vi "UI-BaseParamSet.vi"(8 "error in (no error)":errorcluster caption="错误输入（无错误）") -> (0 "error out":errorcluster caption="错误输出")   [LabVIEW 2017]
uses:
  Picture/SaveButtom.ctl
  Global System.vi
panel:
  in  "Program Update":bool
  in  "Machine Paramter Save Buttom":T1
  out "system time":string
  in  "选项卡控件":enum32{"BaseParamSet", "OtherParamSet"}(tab)
  in  "条码扫描周期":string
  in  "LoadProgram":string(combo)
  in  "BaseParams Save Buttom":T1
  in  "参数B":string
  in  "参数K":string
  in  "校正像素值":string
  in  "Tolerance Params Save":T1
  in  "单位距离":string
  # "秒"
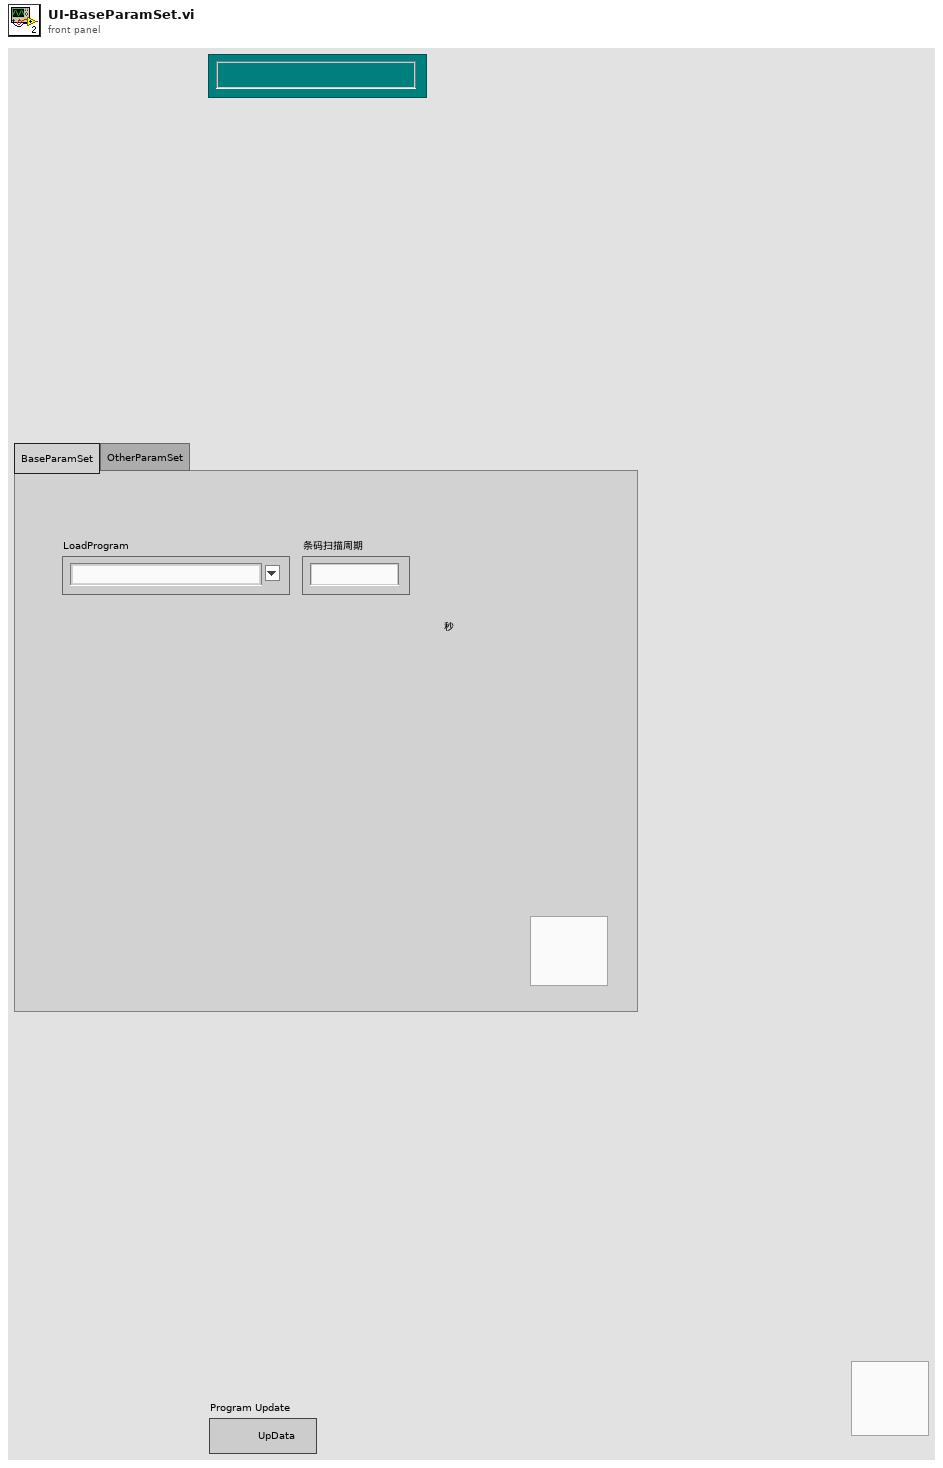
[diagram p1: front panel]
types:
  T1 = typedef "SaveButtom.ctl" = bool
  T2 = cluster{"master data":string, "priority":u16, "secondary data":string[]}
  T3 = cluster{"case name":string[], "queue array":refnum<queue>[]}
  T4 = cluster{"导通气缸上位置":bool, "导通气缸下位置\n":bool, "工位一料到位信号":bool, "工位二料到位信号":bool, "工位三料到位信号":bool, "转盘到位信号":bool, "凸轮感应信号":bool, "导通信号":bool, "真空":bool, "备用":bool, "备用":bool, "备用":bool, "备用":bool, "备用":bool, "备用":bool, "备用":bool, "备用":bool, "备用":bool, "备用":bool, "备用":bool, "备用":bool, "备用":bool, "备用":bool, "备用":bool}
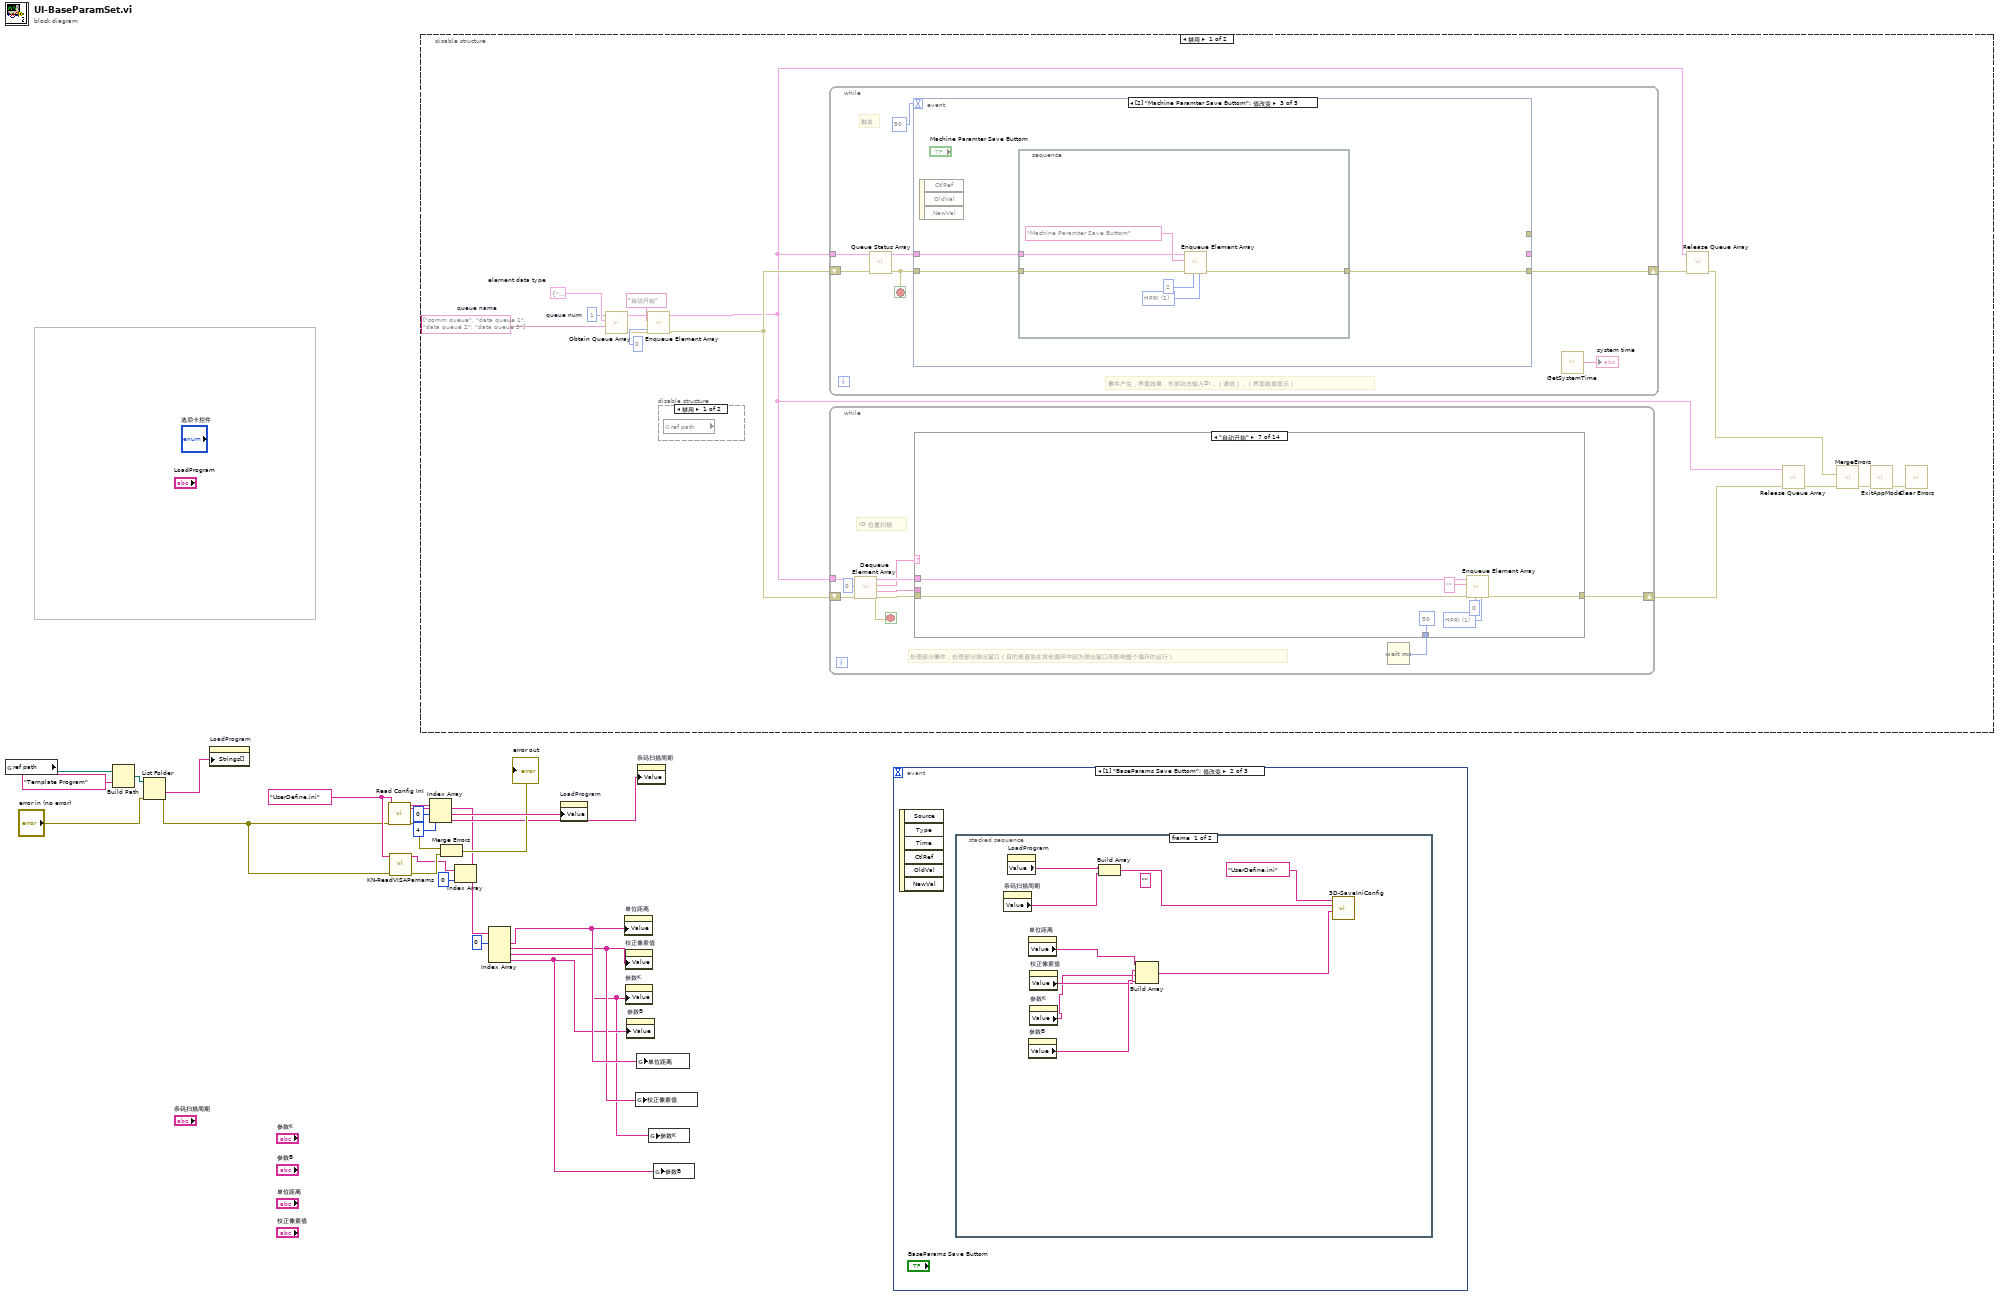
[diagram p0: block diagram]
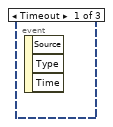
[diagram p2: hidden frame]
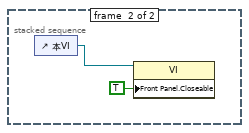
[diagram p3: hidden frame]
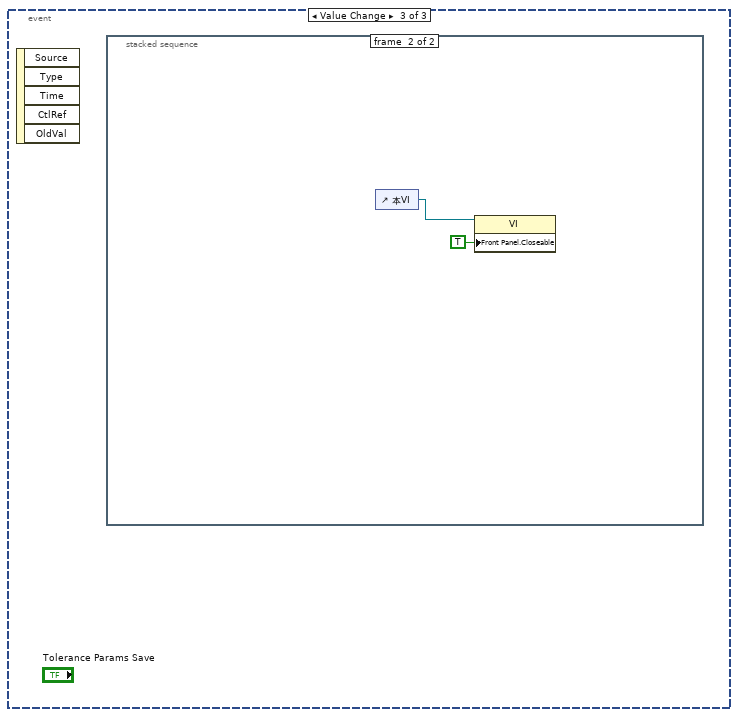
[diagram p4: hidden frame]
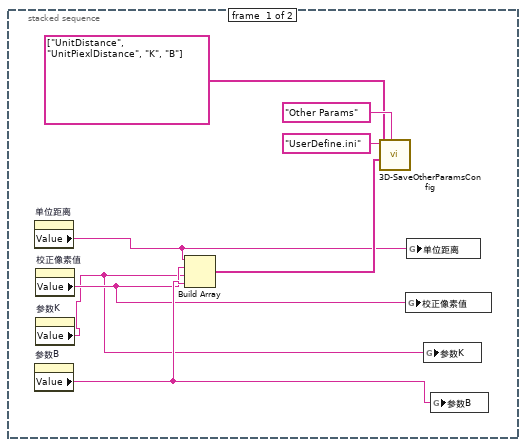
[diagram p5: hidden frame]
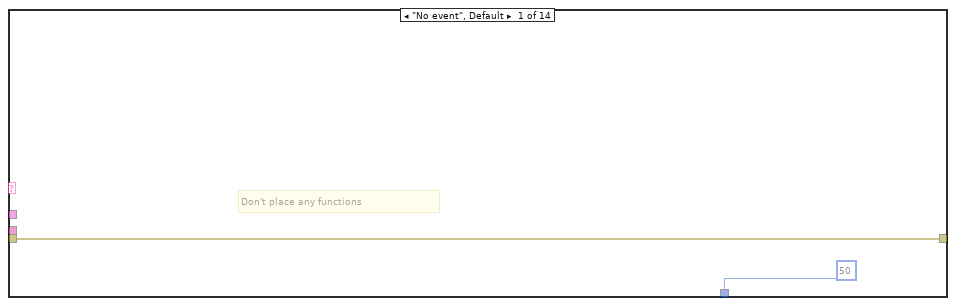
[diagram p7: hidden frame]
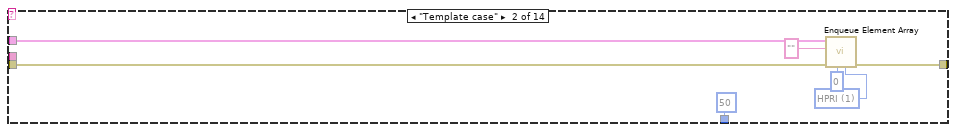
[diagram p8: hidden frame]
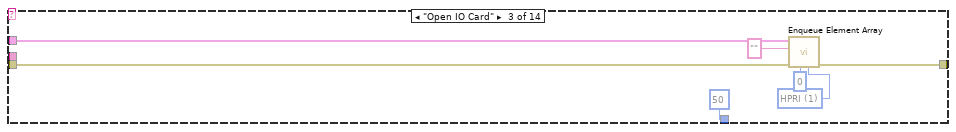
[diagram p9: hidden frame]
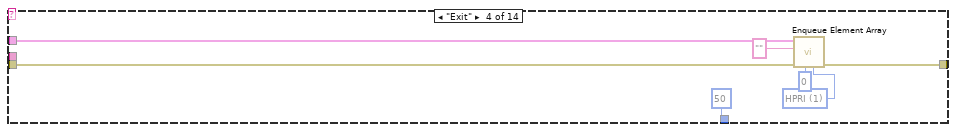
[diagram p10: hidden frame]
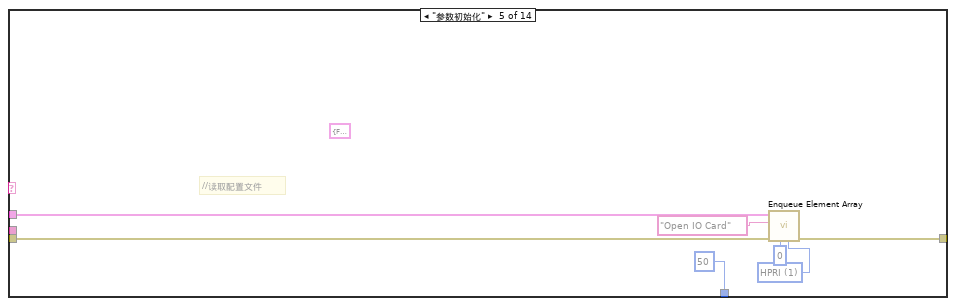
[diagram p11: hidden frame]
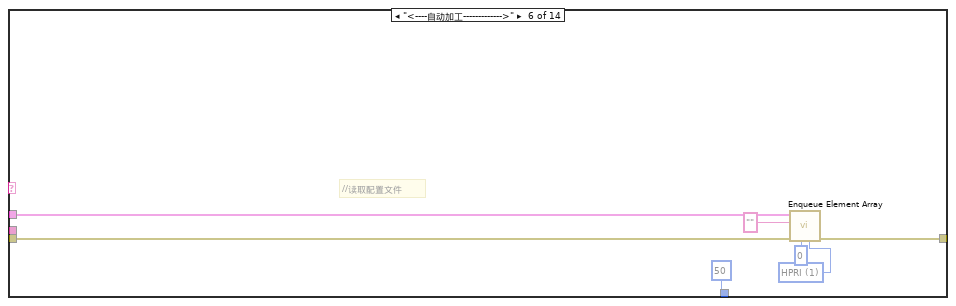
[diagram p12: hidden frame]
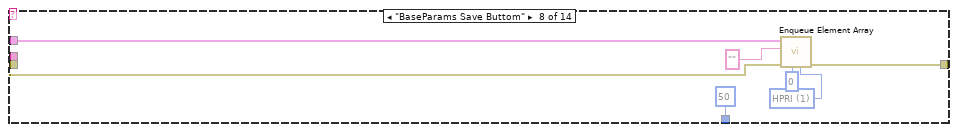
[diagram p13: hidden frame]
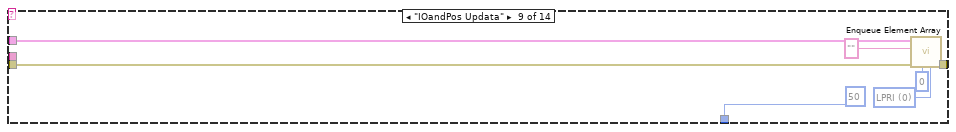
[diagram p14: hidden frame]
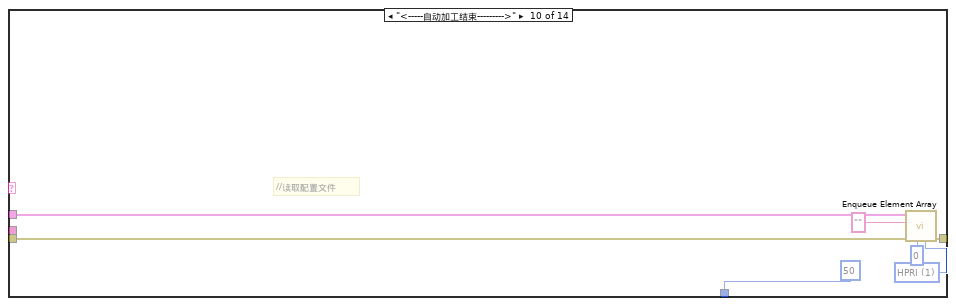
[diagram p15: hidden frame]
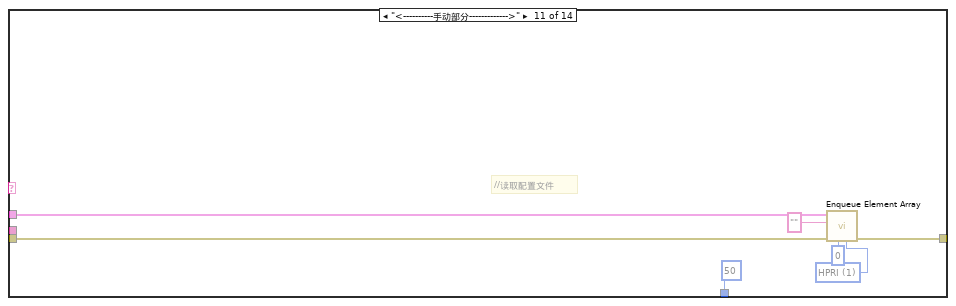
[diagram p16: hidden frame]
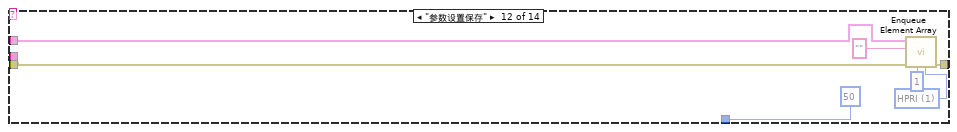
[diagram p17: hidden frame]
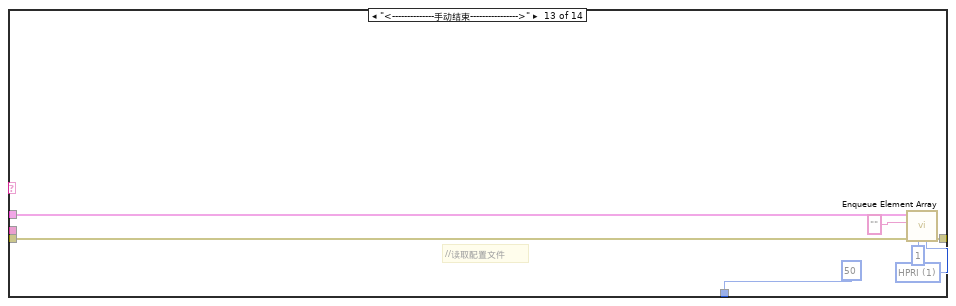
[diagram p18: hidden frame]
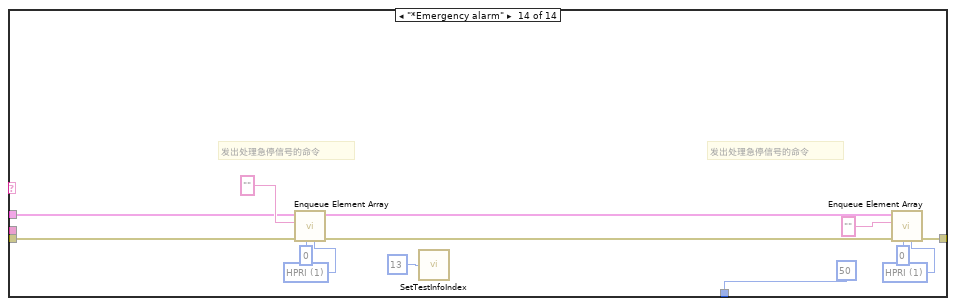
[diagram p19: hidden frame]
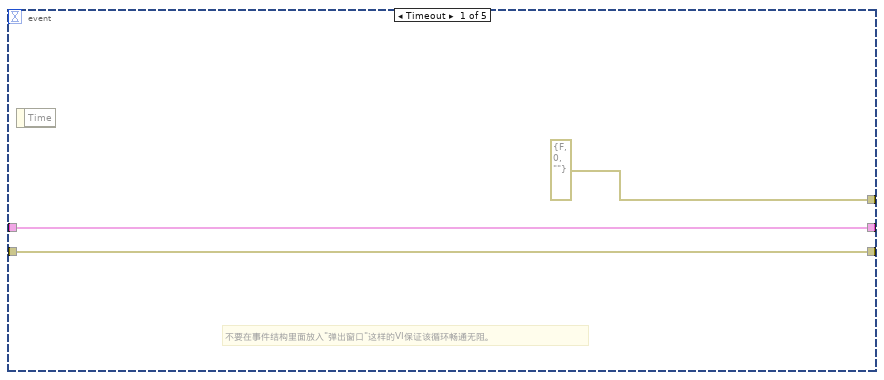
[diagram p20: hidden frame]
diagram:
  w20 = "UserDefine.ini" ("名称或相对路径")
  n1 = global read "Global System.vi" "ref path"() -> (w14:path)
  n2 = Build Path(base path=w14, name or relative path="Template Program" ("名称或相对路径")) -> (appended path=w12:path)
  n3 = List Folder(path=w12, error in="error in (no error)") -> (folder names=w11:string[], error out=w9:errorcluster)  [unwired: 2 in, 2 out]
  n4 = property on="LoadProgram" class="CmbBox"("Strings[]"=w11) -> ()  [unwired: 2 in, 2 out]
  n5 = call "Read Config InI.vi"("名称或相对路径"=w20, "error in (no error)"=w9) -> ("ParamSet"=w22:string[], "Other Params"=w6:string[], "error out"=w19:errorcluster)  [unwired: 13 in, 2 out]
  n6 = call "KN-ReadVISAPamams.vi"("名称或相对路径"=w20, "error in (no error)"=w9) -> ("VISA1 Param"=w16:string[], "error out"=w18:errorcluster)  [unwired: 12 in]
  n7 = disable-structure shown="禁用" {
    frame Disabled {
      w37 = 1  # queue num
      w38 = T2 {"master data"="", "priority"=0, "secondary data"=[]}  # element data type
      w36 = string[] ["comm queue", "data queue 1", "data queue 2", "data queue 3"]  # queue name
      n8 = call "Obtain Queue Array.vi"("queue name"=w36, "element data type"=w38, "queue num"=w37) -> ("error out"=w32:errorcluster, "queue out"=w33:T3)  [unwired: 2 in, 1 out]
      n9 = call "Enqueue Element Array.vi"("queue index"=0, "error in"=w32, "master data"="自动开始", "queue in"=w33) -> ("error out"=w26:errorcluster, "queue out"=w24:T3)  [unwired: 6 in]
      n10 = disable-structure shown="禁用" {
        frame Disabled {
          n11 = global read "Global System.vi" "ref path"() -> ()  [unwired: 1 out]
        }
        frame Enabled {
        }
      }
      n12 = while {
        shift-right: [w147] -> w27
        shift-left: w26 -> [w150]
        tunnel: w24 -> [w152]
        stop <- w148 stop-if-true
        # "触发"
        # "事件产生，界面效果，外部状态输入DI，（通信），（界面数据显示）"
        n13 = call "Queue Status Array.vi"("error in (no error)"=w150, "queue in"=w152) -> ("error out"=w148:errorcluster, "queue out"=w149:T3)  [unwired: 4 in]
        n14 = event shown="[2] \"Machine Paramter Save Buttom\": 值改变" {
          selector: _ -> [_ _ _ _ _]
          dyn-events: _ -> [_ _ _ _ _]
          timeout: 50 -> [_ _ _ _ _]
          tunnel: [errorcluster {"status"=FALSE, "code"=0, "source"=""} ("error out") _ _ _ _] -> _
          tunnel: w149 -> [w155 w163 w167 w176 w188]
          tunnel: w148 -> [w154 w162 w166 w175 w187]
          tunnel: [w154 w161 w165 w174 w186] -> w147
          tunnel: [w155 w160 _ _ _] -> _
          event Timeout {
            # "不要在事件结构里面放入\"弹出窗口\"这样的VI保证该循环畅通无阻。"
            n15 = event-data() -> ()  [unwired: 1 in, 1 out]
          }
          event Panel Close? {
            w158 = u16 1 items=["HPRI"=1, "LPRI"=0] ("priority")
            n16 = event-data() -> ()  [unwired: 1 in, 4 out]
            n17 = call "Enqueue Element Array.vi"("priority"=w158, "queue index"=0, "error in"=w162, "master data"="*Exit application", "queue in"=w163) -> ("error out"=w161:errorcluster, "queue out"=w160:T3)  [unwired: 5 in]
            n18 = event-data("Discard?"=TRUE) -> ()  [unwired: 1 in, 1 out]
          }
          event Value Change {
            n19 = event-data() -> ()  [unwired: 1 in, 3 out]
            n20 = stacked-sequence {
              tunnel: w167 -> [w170]
              tunnel: w166 -> [w169]
              tunnel: [w168] -> w165
              frame #0 {
                w172 = u16 1 items=["HPRI"=1, "LPRI"=0] ("priority")
                n21 = call "Enqueue Element Array.vi"("priority"=w172, "queue index"=2, "error in"=w169, "master data"="Machine Paramter Save Buttom", "queue in"=w170) -> ("error out"=w168:errorcluster)  [unwired: 5 in, 1 out]
              }
            }
          }
          event "Program Update": Value Change {
            n22 = event-data() -> ()  [unwired: 1 in, 6 out]
            n23 = stacked-sequence {
              tunnel: w176 -> [w179]
              tunnel: w175 -> [w178]
              tunnel: [w177] -> w174
              frame #0 {
                w181 = u16 1 items=["HPRI"=1, "LPRI"=0] ("priority")
                n24 = call "Enqueue Element Array.vi"("priority"=w181, "queue index"=2, "error in"=w178, "master data"="Program Update", "queue in"=w179) -> ("error out"=w177:errorcluster)  [unwired: 5 in, 1 out]
              }
            }
          }
          event Value Change {
            w184 = u16 1 items=["HPRI"=1, "LPRI"=0] ("priority")
            n25 = event-data() -> ()  [unwired: 1 in, 3 out]
            n26 = call "Enqueue Element Array.vi"("priority"=w184, "queue index"=0, "error in"=w187, "master data"="BaseParams Save Buttom", "queue in"=w188) -> ("error out"=w186:errorcluster)  [unwired: 5 in, 1 out]
          }
        }
        n27 = call "GetSystemTime.vi"() -> ("date/time string"=→"system time":string)  [unwired: 7 in]
      }
      n28 = while {
        shift-right: [w47] -> w25
        shift-left: w26 -> [w45]
        tunnel: w24 -> [w41]
        stop <- w40 stop-if-true
        # "IO 位置扫描"
        # "处理部分事件；处理部分弹出窗口（目的是避免在其他循环中因为弹出窗口而影响整个循环的运行）"
        n29 = call "Dequeue Element Array.vi"("queue in"=w41, "queue index"=0, "error in"=w45) -> ("queue out"=w44:T3, "master data"=w43:string, "secondary data"=w42:string[], "error out"=w40:errorcluster)  [unwired: 2 in, 1 out]
        n30 = case shown="\"自动开始\"" w43 {
          tunnel: w44 -> [_ w55 w62 w69 w76 w83 w85 w97 w104 w111 w118 w125 w132 w138]
          tunnel: w40 -> [w49 w52 w59 w66 w73 w80 w88 w94 w99 w108 w115 w122 w129 w135]
          tunnel: [w49 w54 w61 w68 w75 w82 w90 w96 w103 w110 w117 w124 w131 w145] -> w47
          tunnel: [50 50 50 50 50 50 50 50 50 50 50 50 50 50] -> w46
          tunnel: w42 -> [_ _ _ _ _ _ _ _ _ _ _ _ _ _]
          frame "No event", Default {
            # "Don't place any functions"
          }
          frame "Template case" {
            w50 = u16 1 items=["HPRI"=1, "LPRI"=0] ("priority")
            n31 = call "Enqueue Element Array.vi"("priority"=w50, "queue index"=0, "error in"=w52, "master data"="" ("Element 1"), "queue in"=w55) -> ("error out"=w54:errorcluster)  [unwired: 5 in, 1 out]
          }
          frame "Open IO Card" {
            w57 = u16 1 items=["HPRI"=1, "LPRI"=0] ("priority")
            n32 = call "Enqueue Element Array.vi"("priority"=w57, "queue index"=0, "error in"=w59, "master data"="" ("Element 1"), "queue in"=w62) -> ("error out"=w61:errorcluster)  [unwired: 5 in, 1 out]
          }
          frame "Exit" {
            w64 = u16 1 items=["HPRI"=1, "LPRI"=0] ("priority")
            n33 = call "Enqueue Element Array.vi"("priority"=w64, "queue index"=0, "error in"=w66, "master data"="" ("Element 1"), "queue in"=w69) -> ("error out"=w68:errorcluster)  [unwired: 5 in, 1 out]
          }
          frame "参数初始化" {
            (unwired) T4 {"导通气缸上位置"=FALSE, "导通气缸下位置\n"=FALSE, "工位一料到位信号"=FALSE, "工位二料到位信号"=FALSE, "工位三料到位信号"=FALSE, "转盘到位信号"=FALSE, "凸轮感应信号"=FALSE, "导通信号"=FALSE, "真空"=FALSE, "备用"=FALSE, "备用"=FALSE, "备用"=FALSE, "备用"=FALSE, "备用"=FALSE, "备用"=FALSE, "备用"=FALSE, "备用"=FALSE, "备用"=FALSE, "备用"=FALSE, "备用"=FALSE, "备用"=FALSE, "备用"=FALSE, "备用"=FALSE, "备用"=FALSE} ("7230 设备DO")
            w71 = u16 1 items=["HPRI"=1, "LPRI"=0] ("priority")
            # "//读取配置文件"
            n34 = call "Enqueue Element Array.vi"("priority"=w71, "queue index"=0, "error in"=w73, "master data"="Open IO Card" ("Element 1"), "queue in"=w76) -> ("error out"=w75:errorcluster)  [unwired: 5 in, 1 out]
          }
          frame "<----自动加工------------->" {
            w78 = u16 1 items=["HPRI"=1, "LPRI"=0] ("priority")
            # "//读取配置文件"
            n35 = call "Enqueue Element Array.vi"("priority"=w78, "queue index"=0, "error in"=w80, "master data"="" ("Element 1"), "queue in"=w83) -> ("error out"=w82:errorcluster)  [unwired: 5 in, 1 out]
          }
          frame "自动开始" {
            w86 = u16 1 items=["HPRI"=1, "LPRI"=0] ("priority")
            n36 = call "Enqueue Element Array.vi"("priority"=w86, "queue index"=0, "error in"=w88, "master data"="" ("Element 1"), "queue in"=w85) -> ("error out"=w90:errorcluster)  [unwired: 5 in, 1 out]
          }
          frame "BaseParams Save Buttom" {
            w92 = u16 1 items=["HPRI"=1, "LPRI"=0] ("priority")
            n37 = call "Enqueue Element Array.vi"("priority"=w92, "queue index"=0, "error in"=w94, "master data"="" ("Element 1"), "queue in"=w97) -> ("error out"=w96:errorcluster)  [unwired: 5 in, 1 out]
          }
          frame "IOandPos Updata" {
            w101 = u16 0 items=["HPRI"=1, "LPRI"=0] ("priority")
            n38 = call "Enqueue Element Array.vi"("priority"=w101, "queue index"=0, "error in"=w99, "master data"="", "queue in"=w104) -> ("error out"=w103:errorcluster)  [unwired: 5 in, 1 out]
          }
          frame "<-----自动加工结束--------->" {
            w106 = u16 1 items=["HPRI"=1, "LPRI"=0] ("priority")
            # "//读取配置文件"
            n39 = call "Enqueue Element Array.vi"("priority"=w106, "queue index"=0, "error in"=w108, "master data"="" ("Element 1"), "queue in"=w111) -> ("error out"=w110:errorcluster)  [unwired: 5 in, 1 out]
          }
          frame "<----------手动部分------------->" {
            w113 = u16 1 items=["HPRI"=1, "LPRI"=0] ("priority")
            # "//读取配置文件"
            n40 = call "Enqueue Element Array.vi"("priority"=w113, "queue index"=0, "error in"=w115, "master data"="" ("Element 1"), "queue in"=w118) -> ("error out"=w117:errorcluster)  [unwired: 5 in, 1 out]
          }
          frame "参数设置保存" {
            w120 = u16 1 items=["HPRI"=1, "LPRI"=0] ("priority")
            n41 = call "Enqueue Element Array.vi"("priority"=w120, "queue index"=1, "error in"=w122, "master data"="" ("Element 1"), "queue in"=w125) -> ("error out"=w124:errorcluster)  [unwired: 5 in, 1 out]
          }
          frame "<--------------手动结束---------------->" {
            w127 = u16 1 items=["HPRI"=1, "LPRI"=0] ("priority")
            # "//读取配置文件"
            n42 = call "Enqueue Element Array.vi"("priority"=w127, "queue index"=1, "error in"=w129, "master data"="" ("Element 1"), "queue in"=w132) -> ("error out"=w131:errorcluster)  [unwired: 5 in, 1 out]
          }
          frame "*Emergency alarm" {
            w141 = u16 1 items=["HPRI"=1, "LPRI"=0] ("priority")
            w142 = u16 1 items=["HPRI"=1, "LPRI"=0] ("priority")
            # "发出处理急停信号的命令"
            # "发出处理急停信号的命令"
            n43 = call "Enqueue Element Array.vi"("priority"=w141, "queue index"=0, "error in"=w135, "master data"="" ("Element 1"), "queue in"=w138) -> ("error out"=w136:errorcluster, "queue out"=w137:T3)  [unwired: 5 in]
            n44 = call "SetTestInfoIndex.vi"("test info index"=13) -> ()
            n45 = call "Enqueue Element Array.vi"("priority"=w142, "queue index"=0, "error in"=w136, "master data"="" ("Element 1"), "queue in"=w137) -> ("error out"=w145:errorcluster)  [unwired: 5 in, 1 out]
          }
        }
        n46 = Wait (ms)(milliseconds to wait=w46) -> ()  [unwired: 1 out]
      }
      n47 = call "Release Queue Array.vi"("error in"=w27, "queue in"=w24) -> ("error out"=w29:errorcluster)  [unwired: 2 in, 3 out]
      n48 = call "Release Queue Array.vi"("error in"=w25, "queue in"=w24) -> ("error out"=w31:errorcluster)  [unwired: 2 in, 3 out]
      n49 = call "MergeErrors.vi"("error in 2 (no error)"=w29, "error in 4 (no error)"=w31) -> ("error out"=w30:errorcluster)  [unwired: 6 in]
      n50 = call "ExitAppMode.vi"("error in (no error)"=w30) -> ("error out"=w28:errorcluster)  [unwired: 10 in]
      n51 = call <vilib>:"Clear Errors.vi"("error in (no error)"=w28) -> ()  [unwired: 5 in, 2 out]
    }
    frame Enabled {
    }
  }
  n52 = Index Array(array=w22, index #1=0 ("索引"), index #2=4 ("索引")) -> (element #1=w21:string, element #2=w7:string)
  n53 = Merge Errors(w19, w18) -> (→"error out":errorcluster)
  n54 = Index Array(array=w16, index=0 ("索引")) -> ()  [unwired: 1 out]
  n55 = Index Array(array=w6, index #1=0 ("索引")) -> (element #1=w4:string, element #2=w3:string, element #3=w1:string, element #4=w2:string)  [unwired: 3 in]
  n56 = property on="LoadProgram" class="CmbBox"("Value"=w21) -> ()  [unwired: 2 in, 2 out]
  n57 = property on="单位距离" class="Str"("Value"=w4) -> ()  [unwired: 2 in, 2 out]
  n58 = property on="校正像素值" class="Str"("Value"=w3) -> ()  [unwired: 2 in, 2 out]
  n59 = property on="参数K" class="Str"("Value"=w1) -> ()  [unwired: 2 in, 2 out]
  n60 = property on="参数B" class="Str"("Value"=w2) -> ()  [unwired: 2 in, 2 out]
  n61 = global write "Global System.vi" "校正像素值"(w3) -> ()
  n62 = global write "Global System.vi" "单位距离"(w4) -> ()
  n63 = property on="条码扫描周期" class="Str"("Value"=w7) -> ()  [unwired: 2 in, 2 out]
  n64 = global write "Global System.vi" "参数K"(w1) -> ()
  n65 = global write "Global System.vi" "参数B"(w2) -> ()
  n66 = event shown="[1] \"BaseParams Save Buttom\": 值改变" {
    selector: _ -> [_ _ _]
    dyn-events: _ -> [_ _ _]
    timeout: _ -> [_ _ _]
    event Timeout {
      n67 = event-data() -> ()  [unwired: 1 in, 3 out]
    }
    event Value Change {
      n68 = event-data() -> ()  [unwired: 1 in, 6 out]
      n69 = stacked-sequence {
        frame #0 {
          (unwired) ""
          n70 = property on="条码扫描周期" class="Str"() -> ("Value"=w194:string)  [unwired: 2 in, 2 out]
          n71 = property on="LoadProgram" class="CmbBox"() -> ("Value"=w196:string)  [unwired: 2 in, 2 out]
          n72 = property on="单位距离" class="Str"() -> ("Value"=w193:string)  [unwired: 2 in, 2 out]
          n73 = property on="参数B" class="Str"() -> ("Value"=w192:string)  [unwired: 2 in, 2 out]
          n74 = property on="校正像素值" class="Str"() -> ("Value"=w191:string)  [unwired: 2 in, 2 out]
          n75 = property on="参数K" class="Str"() -> ("Value"=w190:string)  [unwired: 2 in, 2 out]
          n76 = Build Array(w196, w194) -> (w195:string[])
          n77 = Build Array(w193, w191, w190, w192) -> (w189:string[])
          n78 = call "3D-SaveIniConfig.vi"("VISA1"=w189, "Inputs_BaseParam"=w195, "名称或相对路径"="UserDefine.ini") -> ()  [unwired: 9 in]
        }
        frame #1 {
          n79 = control-ref of="本VI"() -> (w199:refnum<vi>)
          n80 = property class="VI"(reference=w199, "Front Panel.Closeable"=TRUE ("前面板窗口:可关闭")) -> ()  [unwired: 1 in, 2 out]
        }
      }
    }
    event Value Change {
      n81 = event-data() -> ()  [unwired: 1 in, 5 out]
      n82 = stacked-sequence {
        frame #0 {
          n83 = property on="单位距离" class="Str"() -> ("Value"=w203:string)  [unwired: 2 in, 2 out]
          n84 = property on="参数B" class="Str"() -> ("Value"=w202:string)  [unwired: 2 in, 2 out]
          n85 = property on="校正像素值" class="Str"() -> ("Value"=w201:string)  [unwired: 2 in, 2 out]
          n86 = property on="参数K" class="Str"() -> ("Value"=w200:string)  [unwired: 2 in, 2 out]
          n87 = Build Array(w203, w201, w200, w202) -> (w204:string[])
          n88 = call "3D-SaveOtherParamsConfig.vi"("section"="Other Params", "Values"=w204, "Keys"=string[] ["UnitDistance", "UnitPiexlDistance", "K", "B"], "名称或相对路径"="UserDefine.ini") -> ()  [unwired: 8 in]
          n89 = global write "Global System.vi" "校正像素值"(w201) -> ()
          n90 = global write "Global System.vi" "单位距离"(w203) -> ()
          n91 = global write "Global System.vi" "参数K"(w200) -> ()
          n92 = global write "Global System.vi" "参数B"(w202) -> ()
        }
        frame #1 {
          n93 = control-ref of="本VI"() -> (w209:refnum<vi>)
          n94 = property class="VI"(reference=w209, "Front Panel.Closeable"=TRUE ("前面板窗口:可关闭")) -> ()  [unwired: 1 in, 2 out]
        }
      }
    }
  }
